vi "test_Bitpacked Scalar Input.vi"(8 "error in (no error)":errorcluster, 11 "TestCase in":refnum<class "FPGA Addon Scalar Bitpacking Unit Tests.lvclass">) -> (0 "error out":errorcluster, 3 "TestCase out":refnum<class "FPGA Addon Scalar Bitpacking Unit Tests.lvclass">)   [LabVIEW 2018, in "FPGA Addon Scalar Bitpacking Unit Tests.lvclass"]
uses:
  FPGA Addon Scalar Bitpacking Unit Tests.lvclass
  FPGA Addon Scalar Bitpacking Unit Tests.lvclass/FPGA Addon Scalar Bitpacking Unit Tests.ctl
  Addon/Addon Shared/SubVIs/Constants.vi
  <vilib>/NI/NI VeriStand Advanced SysDef API/_SubVIs/SysDef.Search.GUID.vi
  <vilib>/NI/NI VeriStand Advanced SysDef API/_SubVIs/SysDef.Search.GUIDs.vi
  <vilib>/addons/_JKI Toolkits/VI Tester/TestCase.llb/TestCase.lvclass
  Addon/Addon System Explorer/FPGA Addon System Explorer.lvlib
  <vilib>/NI/NI VeriStand Advanced SysDef API/SysDef API/Advanced System Definition.lvlib
  Addon/Addon Shared/FPGA Addon Shared.lvlib
  C:/Program Files (x86)/National Instruments/LabVIEW 2018/vi.lib/addons/_JKI Toolkits/VI Tester/TestCase.llb/TestCase.lvclass
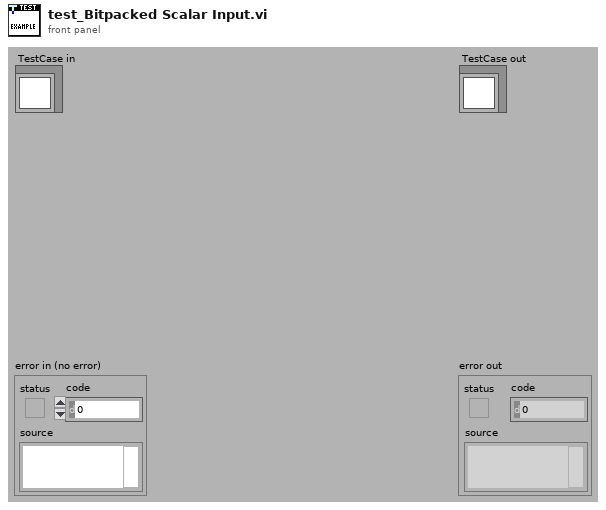
[diagram p1: front panel]
types:
  T1 = typedef "Advanced System Definition.lvlib/TreeItem.Info.ctl" = cluster{"Name":string, "Description":string, "GUID":string, "Is Channel":bool, "Channel":T2, "Is Waveform":bool, "Waveform":T4}
  T2 = typedef "Custom Device API.lvlib/Custom Device Channel.ctl" = cluster{"Type":T3, "Units":string, "Default Value":dbl, "Faultable":bool, "Scalable":bool}
  T3 = typedef "Custom Device API.lvlib/Custom Device Channel Type.ctl" = enum16{"Input", "Output"}
  T4 = typedef "Custom Device API.lvlib/Custom Device Waveform.ctl" = cluster{"Data Type":T5, "Units":string}
  T5 = typedef "Custom Device API.lvlib/Custom Device Waveform DataType.ctl" = enum16{"Double", "Complex Double"}
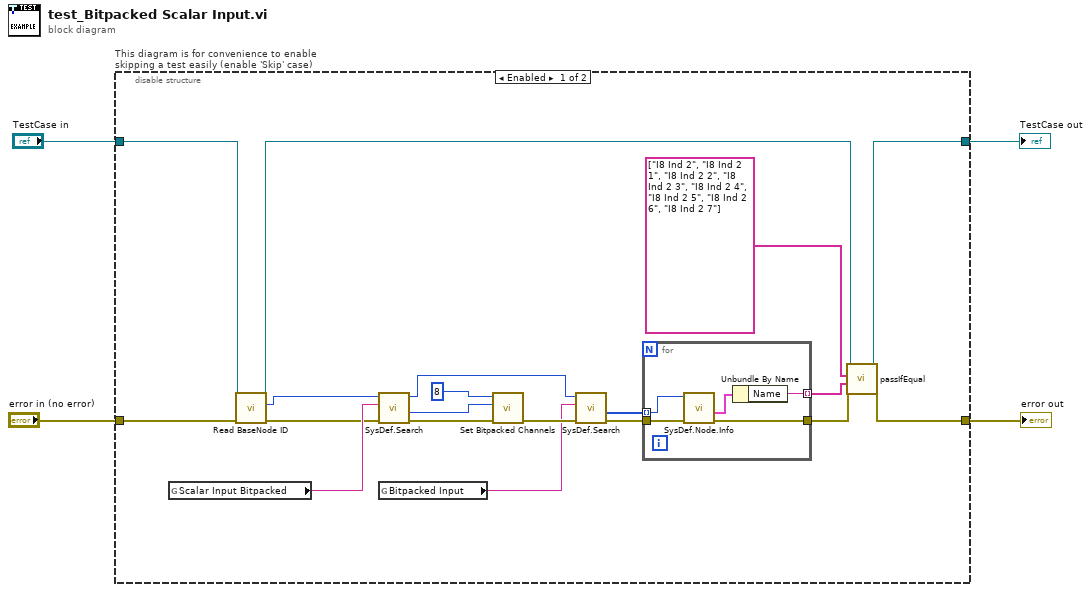
[diagram p0: block diagram]
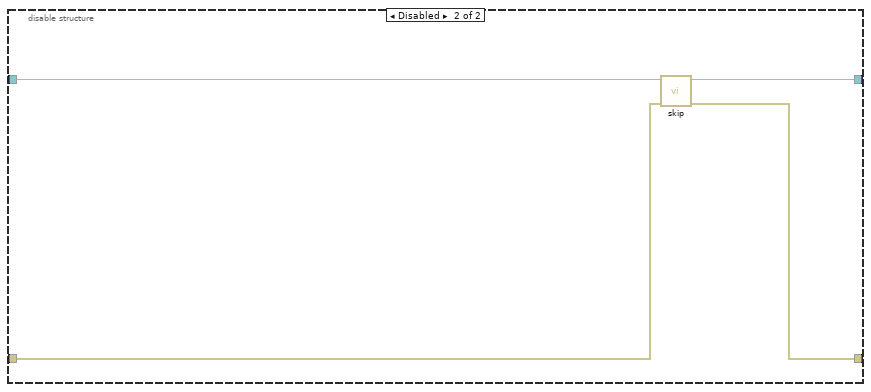
[diagram p2: hidden frame]
diagram:
  n1 = disable-structure "This diagram is for convenience to enable skipping a test easily (enable 'Skip' case)" shown="Enabled" {
    disable-tunnel: "TestCase in" -> [w9 w32]
    disable-tunnel: [w23 w30] -> w1
    disable-tunnel: [w22 w31] -> w3
    disable-tunnel: "error in (no error)" -> [w7 w29]
    frame Enabled {
      n2 = global read "Constants.vi" "Scalar Input Bitpacked"() -> (w16:string)
      n3 = call "Read BaseNode ID.vi"("error in (no error)"=w7, "Scalar Bitpacking Testing in"=w9) -> ("error out"=w6:errorcluster, "BaseNode ID"=w5:u64, "Scalar Bitpacking Testing out"=w8:refnum<class "FPGA Addon Scalar Bitpacking Unit Tests.lvclass">)  [unwired: 7 in]
      n4 = call-poly <vilib>:"SysDef.Search.vi"("error in (no error)"=w6, "GUID"=w16, "nodeID"=w5) -> ("error out"=w20:errorcluster, "Value out"=w19:u64, "nodeID out"=w17:u64)  [unwired: 5 in, 1 out]
      n5 = global read "Constants.vi" "Bitpacked Input"() -> (w15:string)
      n6 = call "Set Bitpacked Channels.vi"("error in (no error)"=w20, "Item Ref in"=w19, "Number of Channels"=u8 8) -> ("error out"=w18:errorcluster)  [unwired: 8 in]
      n7 = call-poly <vilib>:"SysDef.Search.vi"("error in (no error)"=w18, "GUID"=w15, "nodeID"=w17) -> ("error out"=w14:errorcluster, "Values Out"=w13:u64[])  [unwired: 5 in, 2 out]
      n8 = for {
        tunnel: w14 -> [w27]
        tunnel: w13 -> [w28] mode=indexing
        tunnel: [w26] -> w12
        tunnel: [w24] -> w11 mode=indexing
        n9 = call <vilib>:"SysDef.Node.Info.vi"("error in (no error)"=w27, "nodeID"=w28) -> ("error out"=w26:errorcluster, "Item Info"=w25:T1)  [unwired: 6 in, 2 out]
        n10 = Unbundle By Name(w25) -> ("Name"=w24:string)
      }
      n11 = call-dynamic "passIfEqual.vi"("error in (no error)"=w12, "y"=w11, "x"=string[] ["I8 Ind 2", "I8 Ind 2 1", "I8 Ind 2 2", "I8 Ind 2 3", "I8 Ind 2 4", "I8 Ind 2 5", "I8 Ind 2 6", "I8 Ind 2 7"] ("Array"), "TestCase in"=w8) -> ("error out"=w22:errorcluster, "TestCase out"=w23:refnum<class "FPGA Addon Scalar Bitpacking Unit Tests.lvclass">)  [unwired: 6 in]
    }
    frame Disabled {
      # "skip test result while test is under development"
      n12 = call <vilib>:"skip.vi"("error in (no error)"=w29, "TestCase in"=w32) -> ("error out"=w31:errorcluster, "TestCase out"=w30:refnum<class "FPGA Addon Scalar Bitpacking Unit Tests.lvclass">)  [unwired: 8 in]
    }
  }
  "error out" <- w3
  "TestCase out" <- w1
